vi "EEG_2022_040_LabView_3.5.vi"() -> ()   [LabVIEW 2022 SP3]
panel:
  out "Temperature History":cluster{ext, "Temperature":dbl}(graph)
  in  "stop":bool
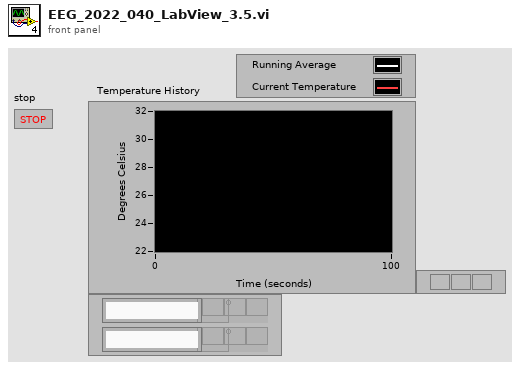
[diagram p1: front panel]
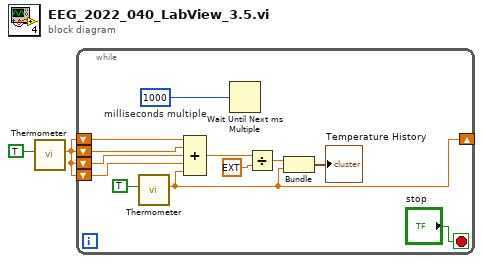
[diagram p0: block diagram]
diagram:
  n1 = call "Thermometer.vi"("Temp Scale"=TRUE) -> ("Temperature"=w2:dbl)  [unwired: 9 in, 1 out]
  n2 = while {
    shift-right: [w4] -> _
    shift-left: w2 -> [w7]
    shift-left: w2 -> [w8]
    shift-left: w2 -> [w9]
    shift-left: w2 -> [w10]
    stop <- "stop" stop-if-true
    w14 = 1000  # milliseconds multiple
    n3 = call "Thermometer.vi"("Temp Scale"=TRUE) -> ("Temperature"=w4:dbl)  [unwired: 9 in, 1 out]
    n4 = Compound Arithmetic op=ADD(w10, w9, w8, w7, w4) -> (w12:dbl)
    n5 = Wait Until Next ms Multiple(millisecond multiple=w14) -> ()  [unwired: 1 out]
    n6 = Divide(x=w12, y=ext 5.0) -> (x/y=w5:ext)
    n7 = Bundle(w5, "Temperature"=w4) -> (→"Temperature History":cluster{ext, "Temperature":dbl})  [unwired: 1 in]
  }
